vi "Set properties lockin.vi"(8 "error in (no error)":errorcluster, 11 "Lockin and Keithley Multimeter in":refnum<class "Lockin and Keithley Multimeter.lvclass">) -> (0 "error out":errorcluster, 3 "Lockin and Keithley Multimeter out":refnum<class "Lockin and Keithley Multimeter.lvclass">)   [LabVIEW 2017, in "Lockin and Keithley Multimeter.lvclass"]
uses:
  Lockin and Keithley Multimeter.lvclass
  Lockin and Keithley Multimeter.lvclass/Lockin and Keithley Multimeter.ctl
  Lockin/sr830/SR830.lvlib
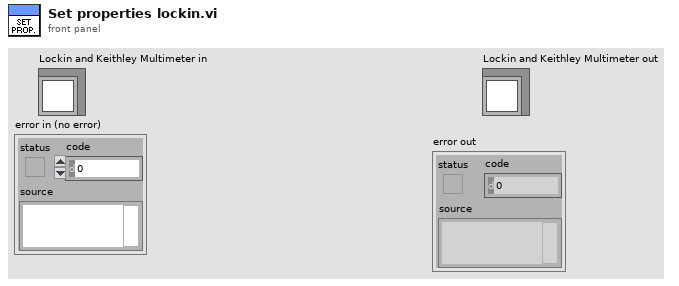
[diagram p1: front panel]
types:
  T1 = typedef "Lockin SR830.lvclass/Sensitivity.ctl" = u16
  T2 = typedef "SR830.lvlib/Tau.ctl" = u16
  T3 = cluster{"error":bool, "code":i32, "source":string}
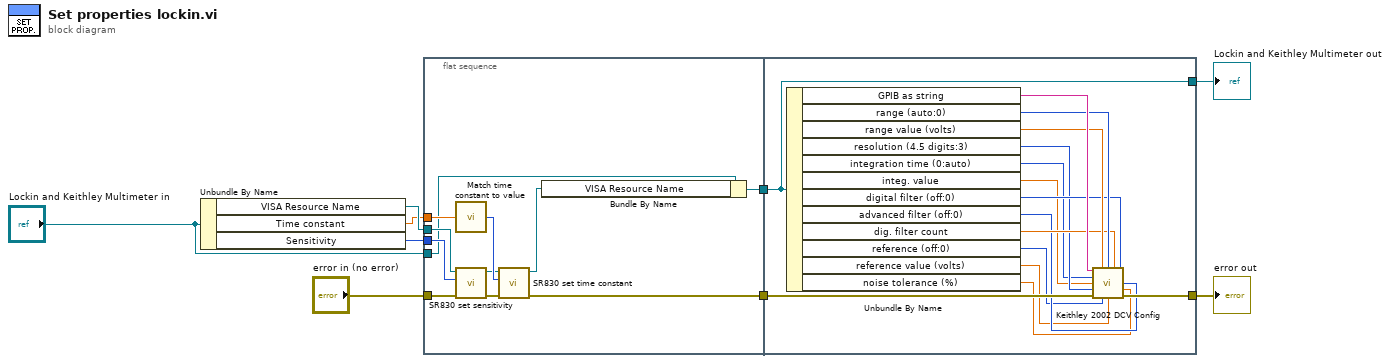
[diagram p0: block diagram]
diagram:
  n1 = Unbundle By Name("Lockin and Keithley Multimeter in") -> ("VISA Resource Name"=w9:refnum<visa-resource-name>, "Time constant"=w7:dbl[unit], "Sensitivity"=w6:T1)
  n2 = flat-sequence {
    tunnel: w9 -> [w20]
    tunnel: "error in (no error)" -> [w19]
    tunnel: w7 -> [w17]
    tunnel: w6 -> [w14]
    tunnel: "Lockin and Keithley Multimeter in" -> [w13]
    tunnel: [w11] -> w3
    tunnel: [w10] -> w2
    tunnel: [w33] -> w4
    tunnel: w3 -> [w33]
    tunnel: w2 -> [w35]
    tunnel: [w34] -> w1
    frame #0 {
      n3 = call "Match time constant to value.vi"("Time constant"=w17) -> ("Tau"=w16:T2)
      n4 = call "SR830 set sensitivity.vi"("error in (no error)"=w19, "Sensitivity"=w14, "VISA resource name"=w20) -> ("error out"=w18:errorcluster, "VISA resource name out"=w15:refnum<visa-resource-name>)  [unwired: 7 in]
      n5 = call "SR830 set time constant.vi"("error in (no error)"=w18, "Tau"=w16, "VISA resource name"=w15) -> ("error out"=w10:errorcluster, "VISA resource name out"=w12:refnum<visa-resource-name>)  [unwired: 7 in]
      n6 = Bundle By Name(cluster=w13, "VISA Resource Name"=w12) -> (w11:refnum<class "Lockin and Keithley Multimeter.lvclass">)
    }
    frame #1 {
      n7 = Unbundle By Name(w33) -> ("GPIB as string"=w32:string, "range (auto:0)"=w30:u16, "range value (volts)"=w31:dbl, "resolution (4.5 digits:3)"=w23:u16, "integration time (0:auto)"=w22:u16, "integ. value"=w21:dbl, "digital filter (off:0)"=w28:u16, "advanced filter (off:0)"=w27:u16, "dig. filter count"=w29:dbl, "reference (off:0)"=w24:u16, "reference value (volts)"=w25:dbl, "noise tolerance (%)"=w26:dbl)
      n8 = call "Keithley 2002 DCV Config.vi"("GPIB address"=w32, "range value (volts)"=w31, "range (auto:0)"=w30, "dig. filter count"=w29, "digital filter (off:0)"=w28, "integration time (0:auto)"=w22, "integ. value"=w21, "advanced filter (off:0)"=w27, "resolution (4.5 digits:3)"=w23, "noise tolerance (%)"=w26, "error in"=w35, "reference (off:0)"=w24, "reference value (volts)"=w25) -> ("error out"=w34:T3)  [unwired: 2 in]
    }
  }
  "Lockin and Keithley Multimeter out" <- w4
  "error out" <- w1
